vi "initialise.vi"(8 "error in (no error)":errorcluster, 11 "GenericPlugin in":refnum<class "SignalWriterMH110203USBStepperMotor.lvclass">) -> (0 "error out":errorcluster, 3 "GenericPlugin out":refnum<class "SignalWriterMH110203USBStepperMotor.lvclass">)   [LabVIEW 2010, in "SignalWriterMH110203USBStepperMotor.lvclass"]
doc: "The dynamic dispatch-version of this VI initalises the plug-in object by allocating and initalising any dynamic resources need."
uses:
  SignalWriterMH110203USBStepperMotor.lvclass
  GenericSignalWriter/GenericSignalWriter/GenericSignalWriter.lvclass
  SignalWriterMH110203USBStepperMotor.lvclass/SignalWriterMH110203USBStepperMotor.ctl
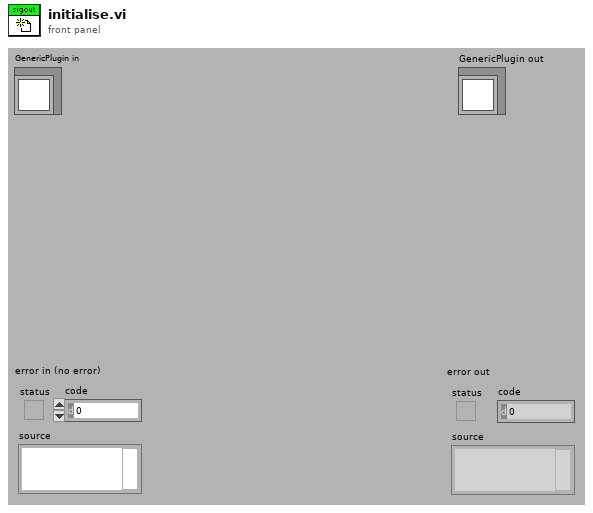
[diagram p1: front panel]
types:
  T1 = typedef "SignalWriterMH110203USBStepperMotor.lvclass/Get State Control (uSMC).ctl" = cluster{"Current Posistion":dbl, "CW/CCW":bool, "Speed":u16, "Temperature":dbl, "Power":u16, "Limit Switch 1":bool, "Limit Switch 2":bool, "After Reset":bool, "Step":u8, "Backlash":bool, "RT Error":bool, "RT State":bool, "Sync In":bool, "Sync Out":bool, "Ext Disconnect":bool, "Usb Powered":bool, "Voltage":dbl, "Working":bool, "SM Position in Encoder Units":i32, "Encoder Current Position":i32}
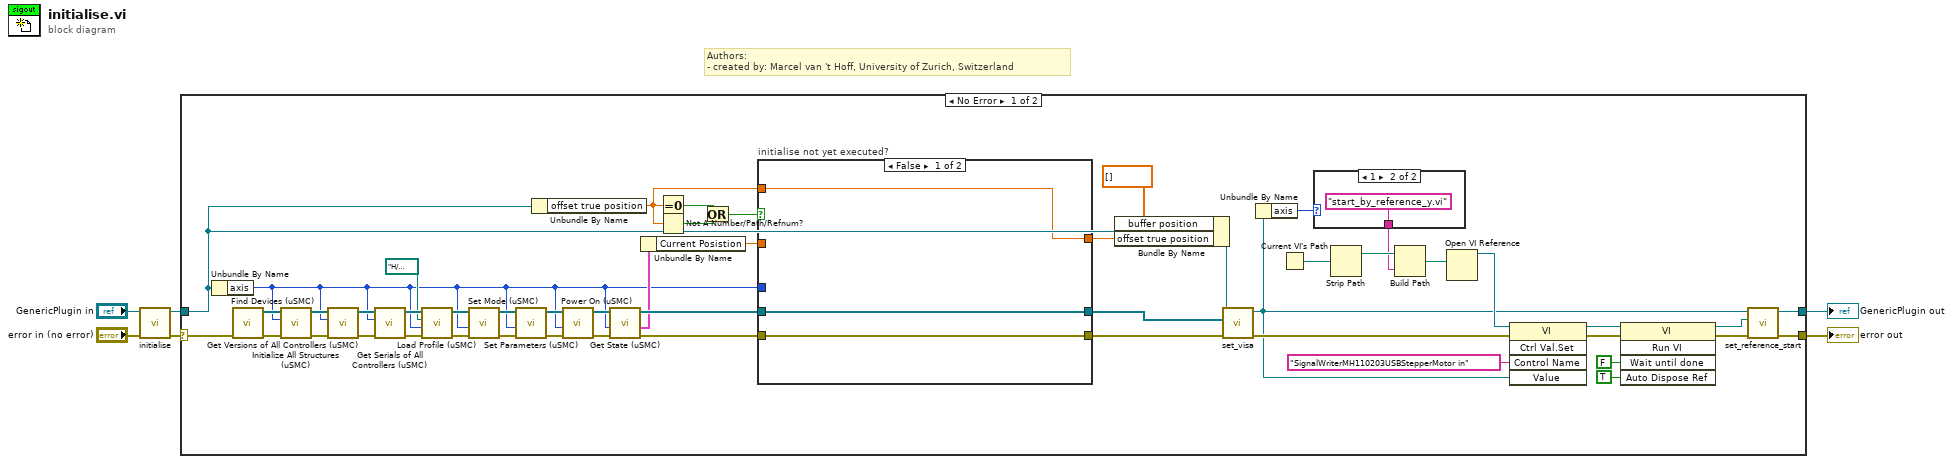
[diagram p0: block diagram]
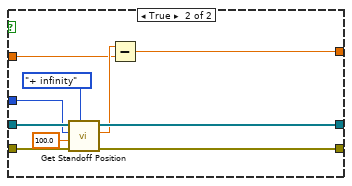
[diagram p2: hidden frame]
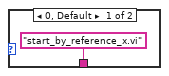
[diagram p3: hidden frame]
diagram:
  # "Authors: \n- created by: Marcel van 't Hoff, University of Zurich, Switzerland"
  n1 = call-parent "initialise.vi"("error in (no error)"="error in (no error)", "GenericPlugin in"="GenericPlugin in") -> ("error out"=w4:errorcluster, "GenericPlugin out"=w2:refnum<class "SignalWriterMH110203USBStepperMotor.lvclass">)  [unwired: 8 in]
  n2 = case shown="No Error" w4 {
    selector: w4 -> [w10 w73]
    tunnel: [w30 w72] -> w3
    tunnel: w2 -> [w8 w72]
    tunnel: [w29 w73] -> w1
    frame No Error {
      n3 = Unbundle By Name(w8) -> ("axis"=w11:i32)
      n4 = call "Find Devices (uSMC).vi"("error in (no error)"=w10) -> ("error out"=w51:errorcluster, "Visa array out"=w52:refnum<visa-resource-name>[])  [unwired: 8 in, 1 out]
      n5 = call "Initialize All Structures (uSMC).vi"("error in"=w51, "axis"=w11, "Visa array in"=w52) -> ("error out"=w55:errorcluster, "Visa array out"=w53:refnum<visa-resource-name>[])  [unwired: 7 in]
      n6 = call "Get Versions of All Controllers (uSMC).vi"("error in"=w55, "axis"=w11, "Visa array in"=w53) -> ("error out"=w56:errorcluster, "Visa array out"=w54:refnum<visa-resource-name>[])  [unwired: 6 in, 1 out]
      n7 = call "Get Serials of All Controllers (uSMC).vi"("error in (no error)"=w56, "axis"=w11, "Visa array in"=w54) -> ("error out"=w50:errorcluster, "Visa array out"=w48:refnum<visa-resource-name>[])  [unwired: 6 in, 1 out]
      n8 = call "Load Profile (uSMC).vi"("error in"=w50, "axis"=w11, "Path"=path "H:/Programming/+ Labview/10 uEye camera/100923/subVI/Standa/Standa_8MR151-1-670mA_D-Sub-15Pin.pre", "Visa array in"=w48) -> ("error out"=w49:errorcluster, "Visa array out"=w47:refnum<visa-resource-name>[])  [unwired: 5 in, 1 out]
      n9 = call "Set Mode (uSMC).vi"("error in (no error)"=w49, "Index"=w11, "Visa Array in"=w47) -> ("error out"=w39:errorcluster, "Visa Array out"=w37:refnum<visa-resource-name>[])  [unwired: 7 in]
      n10 = call "Set Parameters (uSMC).vi"("error in (no error)"=w39, "Index"=w11, "Visa array in"=w37) -> ("error out"=w38:errorcluster, "Visa Array out"=w36:refnum<visa-resource-name>[])  [unwired: 7 in]
      n11 = Unbundle By Name(w8) -> ("offset true position"=w7:dbl)
      n12 = call "Power On (uSMC).vi"("error in (no error)"=w38, "Index"=w11, "Visa Array in"=w36) -> ("error out"=w45:errorcluster, "Visa Array out"=w44:refnum<visa-resource-name>[])  [unwired: 7 in]
      n13 = call "Get State (uSMC).vi"("error in (no error)"=w45, "SM number"=w11, "Visa array in"=w44) -> ("error out"=w34:errorcluster, "State cluster"=w33:T1, "Visa array out"=w35:refnum<visa-resource-name>[])  [unwired: 6 in]
      n14 = Unbundle By Name(w33) -> ("Current Posistion"=w32:dbl)
      n15 = Equal To 0?(x=w7) -> (x = 0?=w13:bool)
      n16 = Not A Number/Path/Refnum?(number/path/refnum=w7) -> (NaN/Path/Refnum?=w12:bool)
      n17 = Or(x=w13, y=w12) -> (x .or. y?=w9:bool)
      n18 = case "initialise not yet executed?" shown="False" w9 {
        tunnel: [w57 w69] -> w43
        tunnel: [w58 w68] -> w41
        tunnel: [w59 w67] -> w40
        tunnel: w35 -> [w59 w64]
        tunnel: w34 -> [w58 w63]
        tunnel: w32 -> [_ w61]
        tunnel: w11 -> [_ w60]
        tunnel: w7 -> [w57 _]
        frame False {
        }
        frame True {
          n19 = call "Get Standoff Position.vi"("Direction"=enum16{"- infinity", "+ infinity"}."+ infinity", "error in (no error)"=w63, "Timeout (sec)"=100.0, "Index"=w60, "Visa Array in"=w64) -> ("error out"=w68:errorcluster, "Standoff"=w62:dbl, "Visa Array out"=w67:refnum<visa-resource-name>[])  [unwired: 3 in, 1 out]
          n20 = Subtract(x=w62, y=w61) -> (x-y=w69:dbl)
        }
      }
      n21 = Bundle By Name(cluster=w8, "buffer position"=dbl[] [], "offset true position"=w43) -> (w42:refnum<class "SignalWriterMH110203USBStepperMotor.lvclass">)
      n22 = call-dynamic "set_visa.vi"("error in (no error)"=w41, "visa array"=w40, "SignalWriterMH110203USBStepperMotor in"=w42) -> ("error out"=w18:errorcluster, "SignalWriterMH110203USBStepperMotor out"=w14:refnum<class "SignalWriterMH110203USBStepperMotor.lvclass">)  [unwired: 7 in]
      n23 = Unbundle By Name(w14) -> ("axis"=w24:i32)
      n24 = Current VI's Path() -> (path=w23:path)
      n25 = case shown="1" w24 {
        tunnel: ["start_by_reference_x.vi" "start_by_reference_y.vi"] -> w20
        frame 0, Default {
        }
        frame 1 {
        }
      }
      n26 = Strip Path(path=w23) -> (stripped path=w22:path)  [unwired: 1 out]
      n27 = Build Path(base path=w22, name or relative path=w20) -> (appended path=w21:path)
      n28 = Open VI Reference(vi path=w21) -> (vi reference=w19:refnum<vi>)  [unwired: 5 in, 1 out]
      n29 = invoke class="VI" method="Ctrl Val.Set"(reference=w19, error in=w18, "Control Name"="SignalWriterMH110203USBStepperMotor in", "Value"=w14) -> (reference out=w16:refnum<vi>, error out=w17:errorcluster)  [unwired: 1 in, 3 out]
      n30 = invoke class="VI" method="Run VI"(reference=w16, error in=w17, "Wait until done"=FALSE ("Wait Until Done"), "Auto Dispose Ref"=TRUE ("Auto Dispose Reference")) -> (reference out=w28:refnum<vi>, error out=w27:errorcluster)  [unwired: 1 in, 3 out]
      n31 = call-dynamic "set_reference_start.vi"("error in (no error)"=w27, "reference start.vi 2"=w28, "SignalWriterMH110203USBStepperMotor in"=w14) -> ("error out"=w29:errorcluster, "SignalWriterMH110203USBStepperMotor out"=w30:refnum<class "SignalWriterMH110203USBStepperMotor.lvclass">)  [unwired: 7 in]
    }
    frame Error {
    }
  }
  "error out" <- w1
  "GenericPlugin out" <- w3
